vi "AlgorithmOptimize.vi"(2 "MatchBallY":dbl, 3 "MatchBallX":dbl, 4 "D2 Y COM":dbl, 5 "D2 X COM":dbl, 6 "D1Y COM":dbl, 7 "D1 X COM 2":dbl) -> (1 "THETA":dbl)   [LabVIEW 2014]
panel:
  out "Angles":dbl[](array[numeric])
  out "max index(es)":i32
  out "max value":dbl
  out "Minimum X separations":dbl[](array[numeric])
  # "theta Calculation"
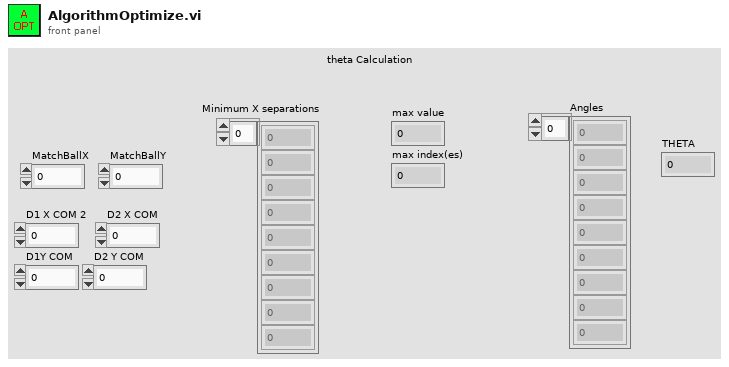
[diagram p1: front panel]
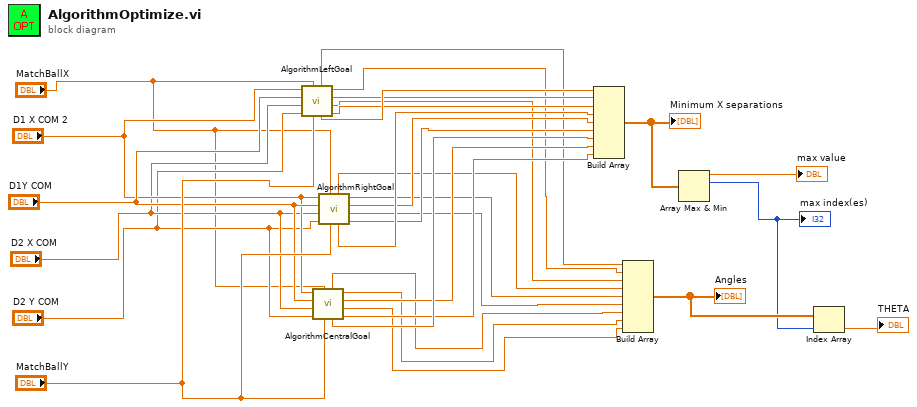
[diagram p0: block diagram]
diagram:
  n1 = call "AlgorithmLeftGoal.vi"("MatchBallY"="MatchBallY", "MatchBallX"="MatchBallX", "D2 Y COM"="D2 Y COM", "D2 X COM"="D2 X COM", "D1Y COM"="D1Y COM", "D1 X COM"="D1 X COM 2") -> ("min x3"=w21:dbl, "aS"=w10:dbl, "min x2"=w22:dbl, "aRW"=w11:dbl, "min x"=w23:dbl, "Theta LG,LW"=w12:dbl)
  n2 = call "AlgorithmCentralGoal.vi"("MatchBallY"="MatchBallY", "MatchBallX"="MatchBallX", "D2 Y COM"="D2 Y COM", "D2 X COM"="D2 X COM", "D1Y COM"="D1Y COM", "D1 X COM"="D1 X COM 2") -> ("min x3"=w15:dbl, "aS"=w4:dbl, "min x2"=w16:dbl, "aRW"=w5:dbl, "min x"=w17:dbl, "Theta LG,LW"=w6:dbl)
  n3 = call "AlgorithmRightGoal.vi"("MatchBallY"="MatchBallY", "MatchBallX"="MatchBallX", "D2 Y COM"="D2 Y COM", "D2 X COM"="D2 X COM", "D1Y COM"="D1Y COM", "D1 X COM"="D1 X COM 2") -> ("min x3"=w18:dbl, "aS"=w7:dbl, "min x2"=w19:dbl, "aRW"=w8:dbl, "min x"=w20:dbl, "Theta LG,LW"=w9:dbl)
  n4 = Build Array(w23, w22, w21, w20, w19, w18, w17, w16, w15) -> (w14:dbl[])
  "Minimum X separations" <- w14
  n5 = Build Array(w12, w11, w10, w9, w8, w7, w6, w5, w4) -> (w3:dbl[])
  "Angles" <- w3
  n6 = Array Max & Min(array=w14) -> (max value=→"max value":dbl, max index (indices)=w2:i32)  [unwired: 2 out]
  "max index(es)" <- w2
  n7 = Index Array(array=w3, index=w2) -> (element=→"THETA":dbl)
